vi "参考-写入数据库.vi"(6 "数据库UDL路径":path, 7 "ROI左上角Y":i32, 8 "ROI左上角X":i32, 9 "框号":dbl format="%#_13g", 10 "Array输入 2":refnum<vi>, 11 "Array输入":refnum<vi>) -> ()   [LabVIEW 2018]
uses:
  <vilib>/addons/database/Connection.llb/DB Tools Open Connec (Path).vi
  <vilib>/addons/database/NI_Database_API.lvlib
  <vilib>/addons/database/Connection.llb/DB Tools Open Connec (String).vi
panel:
  out "分层数据":dbl[][](array[numeric])
  out "弥散数据":dbl[][](array[numeric])
  out "个数":i32
  out "Z值":dbl
  out "tables":string[](array[string])
  out "error out":errorcluster
  out "Connection Succeeded?":bool
  in  "Connection Method":u16(ring) items=["ODBC System DSN", "UDL File", "Prompt"]
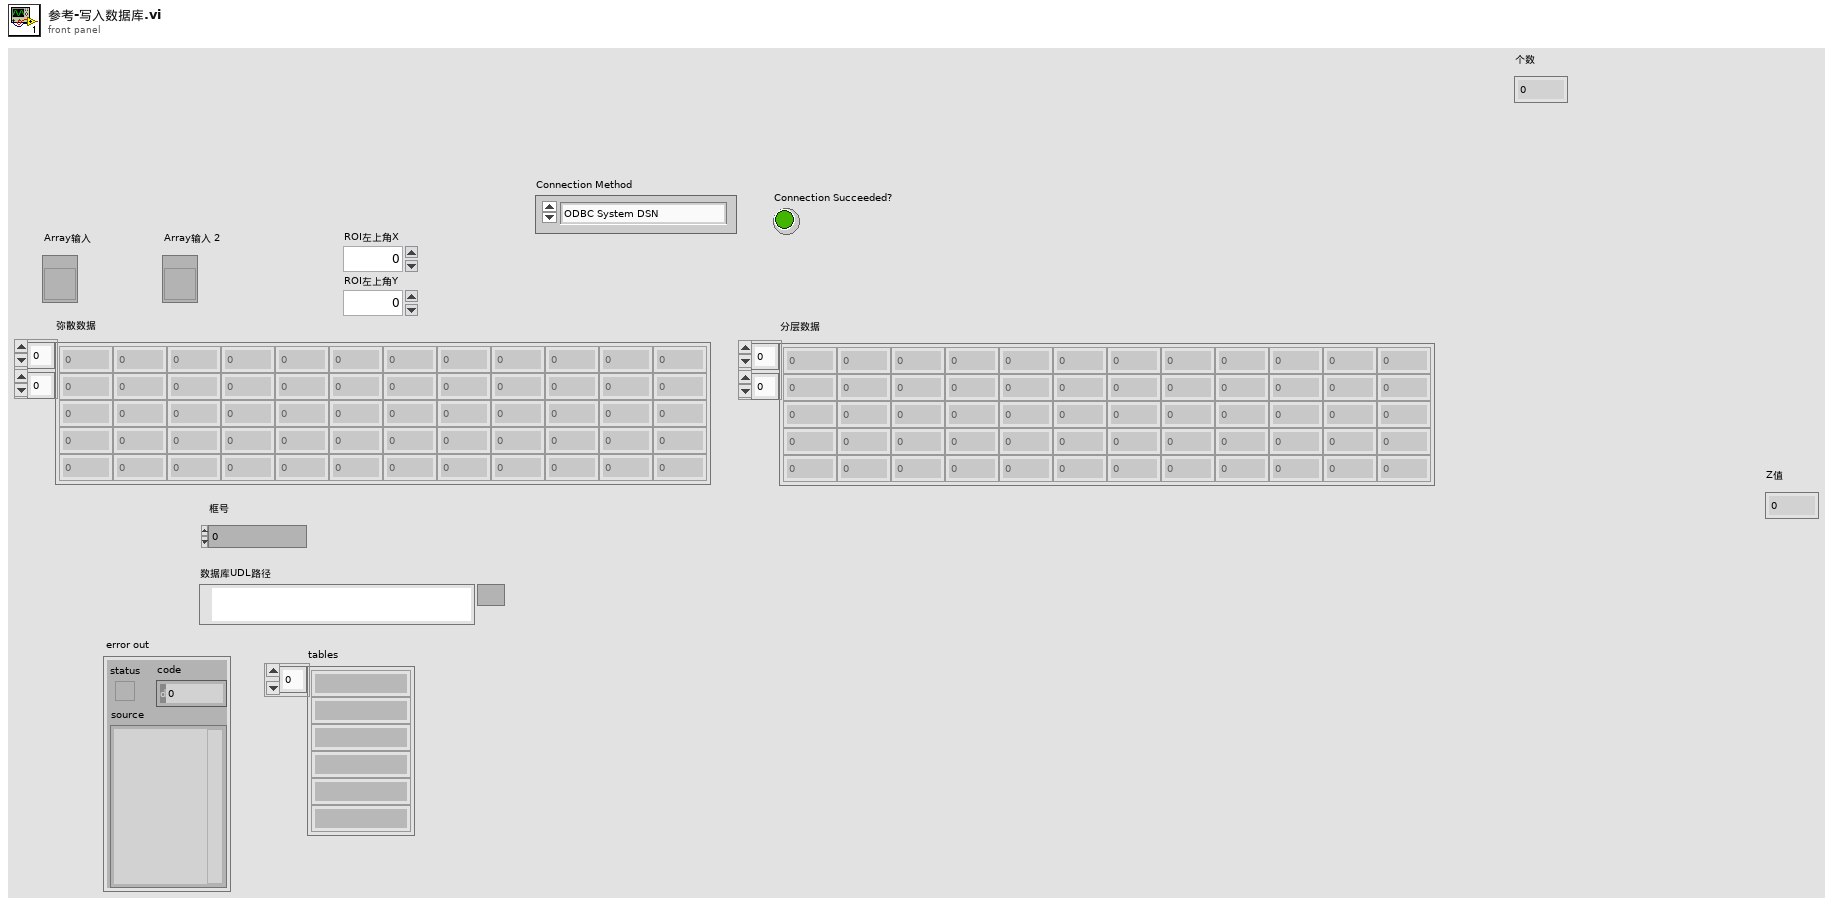
[diagram p1: front panel]
types:
  T1 = typedef "NI_Database_API.lvlib/Conn ObjectReference.ctl" = refnum<k1>
  T2 = cluster{"框号":dbl, "Numeric":dbl, dbl, dbl, "Numeric":dbl, "Numeric":dbl, "Numeric":dbl, "Numeric":dbl, dbl, string}
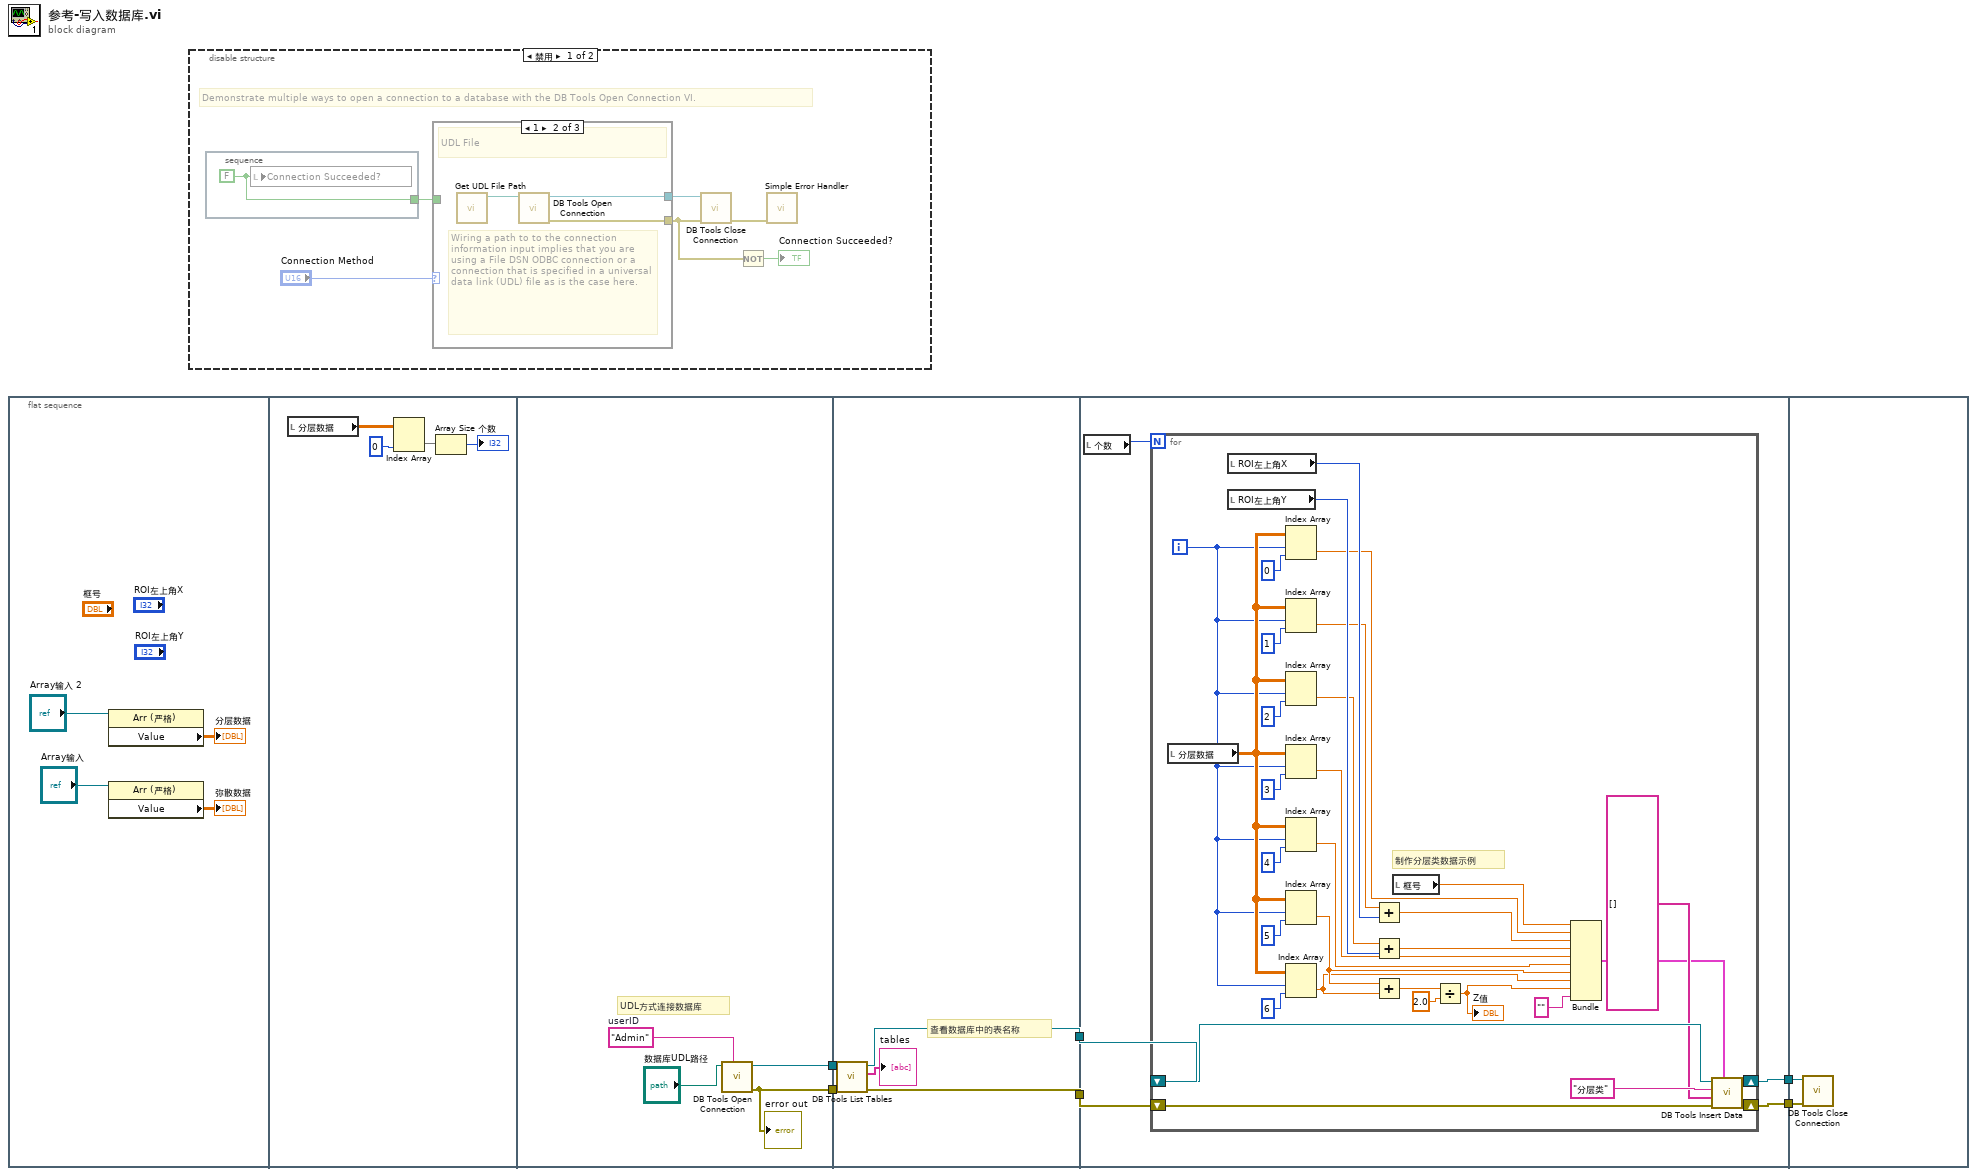
[diagram p0: block diagram]
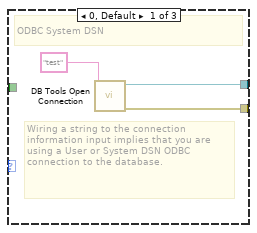
[diagram p2: hidden frame]
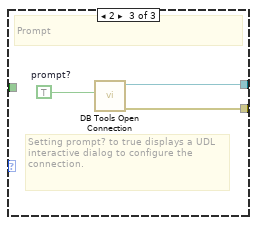
[diagram p3: hidden frame]
diagram:
  n1 = flat-sequence {
    tunnel: [w16] -> w6
    tunnel: [w15] -> w3
    tunnel: w6 -> [w22]
    tunnel: [w21] -> w5
    tunnel: w3 -> [w20]
    tunnel: [w19] -> w2
    tunnel: w5 -> [w28]
    tunnel: [w27] -> w4
    tunnel: w2 -> [w26]
    tunnel: [w25] -> w1
    tunnel: w4 -> [w62]
    tunnel: w1 -> [w61]
    frame #0 {
      n2 = property class="Arr (严格)"(reference="Array输入 2") -> ("Value"=→"分层数据":dbl[][])  [unwired: 1 in, 2 out]
      n3 = property class="Arr (严格)"(reference="Array输入") -> ("Value"=→"弥散数据":dbl[][])  [unwired: 1 in, 2 out]
    }
    frame #1 {
      n4 = local read "分层数据"() -> (w11:dbl[][])
      n5 = Index Array(array=w11, index (col)=0 ("禁用的索引 (列)")) -> (element=w13:dbl[])  [unwired: 1 in]
      n6 = Array Size(array=w13) -> (size(s)=→"个数":i32)
    }
    frame #2 {
      w18 = "Admin"  # userID
      # "UDL方式连接数据库"
      n7 = call-poly <vilib>:"DB Tools Open Connection.vi"("userID"=w18, "connection information"="数据库UDL路径") -> ("error out"=w15:errorcluster, "connection reference"=w16:T1)  [unwired: 6 in]
      "error out" <- w15
    }
    frame #3 {
      # "查看数据库中的表名称"
      n8 = call <vilib>:"DB Tools List Tables.vi"("error in (no error)"=w20, "connection reference"=w22) -> ("error out"=w19:errorcluster, "tables"=→"tables":string[], "connection reference out"=w21:T1)  [unwired: 3 in]
    }
    frame #4 {
      n9 = local read "个数"() -> (w24:i32)
      n10 = for {
        N: w24 -> [_]
        shift-right: [w57] -> w27
        shift-left: w28 -> [w60]
        shift-right: [w55] -> w25
        shift-left: w26 -> [w56]
        i -> [w29]
        # "制作分层类数据示例"
        n11 = local read "分层数据"() -> (w54:dbl[][])
        n12 = local read "ROI左上角X"() -> (w52:i32)
        n13 = local read "ROI左上角Y"() -> (w53:i32)
        n14 = Index Array(array=w54, index (row)=w29, index (col)=0 ("禁用的索引 (列)")) -> (element=w47:dbl)
        n15 = Index Array(array=w54, index (row)=w29, index (col)=1 ("禁用的索引 (列)")) -> (element=w48:dbl)
        n16 = Index Array(array=w54, index (row)=w29, index (col)=2 ("禁用的索引 (列)")) -> (element=w49:dbl)
        n17 = Index Array(array=w54, index (row)=w29, index (col)=3 ("禁用的索引 (列)")) -> (element=w46:dbl)
        n18 = Index Array(array=w54, index (row)=w29, index (col)=4 ("禁用的索引 (列)")) -> (element=w45:dbl)
        n19 = Index Array(array=w54, index (row)=w29, index (col)=5 ("禁用的索引 (列)")) -> (element=w42:dbl)
        n20 = Index Array(array=w54, index (row)=w29, index (col)=6 ("禁用的索引 (列)")) -> (element=w40:dbl)
        n21 = Add(x=w48, y=w52) -> (x+y=w50:dbl)
        n22 = Add(x=w49, y=w53) -> (x+y=w51:dbl)
        n23 = Add(x=w42, y=w40) -> (x+y=w43:dbl)
        n24 = local read "框号"() -> (w44:dbl)
        n25 = Divide(x=w43, y=2.0) -> (x/y=w41:dbl)
        "Z值" <- w41
        n26 = Bundle("框号"=w44, "Numeric"=w47, w50, w51, "Numeric"=w46, "Numeric"=w45, "Numeric"=w42, "Numeric"=w40, w41, "") -> (w30:T2)  [unwired: 1 in]
        n27 = call <vilib>:"DB Tools Insert Data.vi"("data"=w30, "error in (no error)"=w56, "columns"=string[] [], "table"="分层类", "connection reference"=w60) -> ("error out"=w55:errorcluster, "connection reference out"=w57:T1)  [unwired: 5 in]
      }
    }
    frame #5 {
      n28 = call <vilib>:"DB Tools Close Connection.vi"("error in (no error)"=w61, "connection reference"=w62) -> ()  [unwired: 5 in, 1 out]
    }
  }
  n29 = disable-structure shown="禁用" {
    frame Disabled {
      # "Demonstrate multiple ways to open a connection to a database with the DB Tools Open Connection VI."
      n30 = stacked-sequence {
        tunnel: [w69] -> w67
        frame #0 {
          w69 = FALSE ("connection succeeded?")
          n31 = local write "Connection Succeeded?"(w69) -> ()
        }
      }
      n32 = case shown="1" "Connection Method" {
        tunnel: [w71 w74 w78] -> w65
        tunnel: [w70 w75 w77] -> w63
        tunnel: w67 -> [_ _ _]
        frame 0, Default {
          # "Wiring a string to the connection information input implies that you are using a User or System DSN ODBC connection to the database."
          # "ODBC System DSN"
          n33 = call-poly <vilib>:"DB Tools Open Connection.vi"("connection information"="test") -> ("error out"=w70:errorcluster, "connection reference"=w71:T1)  [unwired: 7 in]
        }
        frame 1 {
          # "Wiring a path to to the connection information input implies that you are using a File DSN ODBC connection or a connection that is specified in a universal data link (UDL) file as is the case here."
          # "UDL File"
          n34 = call "Get UDL File Path.vi"() -> ("UDL file path"=w73:path)  [unwired: 11 in]
          n35 = call-poly <vilib>:"DB Tools Open Connection.vi"("connection information"=w73) -> ("error out"=w75:errorcluster, "connection reference"=w74:T1)  [unwired: 7 in]
        }
        frame 2 {
          w76 = TRUE  # prompt?
          # "Setting prompt? to true displays a UDL interactive dialog to configure the connection."
          # "Prompt"
          n36 = call-poly <vilib>:"DB Tools Open Connection.vi"("prompt? (F)"=w76) -> ("error out"=w77:errorcluster, "connection reference"=w78:T1)  [unwired: 7 in]
        }
      }
      n37 = call <vilib>:"DB Tools Close Connection.vi"("error in (no error)"=w63, "connection reference"=w65) -> ("error out"=w66:errorcluster)  [unwired: 5 in]
      n38 = Not(x=w63) -> (.not. x?=→"Connection Succeeded?":bool)
      n39 = call <vilib>:"Simple Error Handler.vi"("error in (no error)"=w66) -> ()  [unwired: 4 in, 5 out]
    }
    frame Enabled {
    }
  }
